vi "RT-Pumb NS reader.vi"(8 "error in (no error)":errorcluster) -> (0 "error IO":errorcluster, 2 "Message Data":variant, 3 "Message":string)   [LabVIEW 2022 SP3]
uses:
  SeCrTs-RT_Global_R.vi
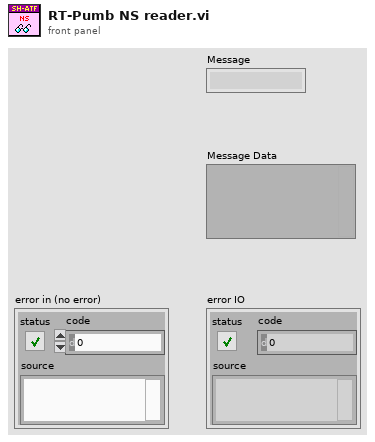
[diagram p1: front panel]
types:
  T1 = cluster{"Message":string, "Message Data":variant}
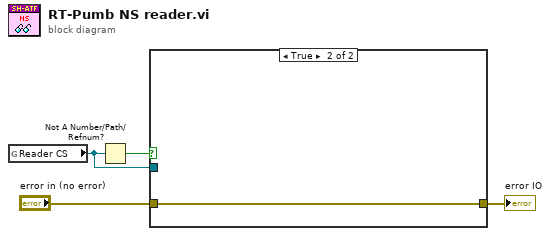
[diagram p0: block diagram]
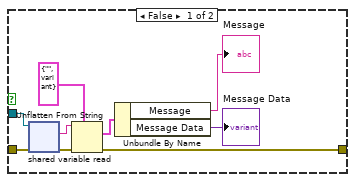
[diagram p2: hidden frame]
diagram:
  n1 = global read "SeCrTs-RT_Global_R.vi" "Reader CS"() -> (w1:refnum<k21>)
  n2 = Not A Number/Path/Refnum?(number/path/refnum=w1) -> (NaN/Path/Refnum?=w3:bool)
  n3 = case shown="True" w3 {
    tunnel: "error in (no error)" -> [w8 w14]
    tunnel: w1 -> [w9 _]
    tunnel: [w5 w14] -> w2
    frame False {
      n4 = shared-variable-read(w9, w8) -> (w6:errorcluster, w7:string)  [unwired: 1 in, 2 out]
      n5 = Unflatten From String(type=T1 {"Message"="", "Message Data"=variant} ("input cluster"), binary string=w7, error in (no error)=w6) -> (value=w10:T1, error out=w5:errorcluster)  [unwired: 2 in, 1 out]
      n6 = Unbundle By Name(w10) -> ("Message"=→"Message":string, "Message Data"=→"Message Data":variant)
    }
    frame True {
    }
  }
  "error IO" <- w2
